vi "mod_Jakes fading profile.vi"(0 "profile length (samples)":i32=1000, 5 "sampling frequency (hz)":dbl=1.0 format="%.2f", 7 "doppler spread (hz)":dbl=1.0 format="%.2f", 9 "seed in (0xFFFFFFFF)":i32=-1 format="%.0x", 11 "error in (no error)":errorcluster, 12 "fading variance":dbl=1.0 format="%.2f", 13 "reset? (T)":bool=TRUE, 14 "number of paths":i32=1) -> (4 "fading profile":cdb[][](array[numeric]) format="%.2f", 10 "next seed":i32 format="%.0x", 15 "error out":errorcluster)   [LabVIEW 2020, in "niDMT.lvlib"]
uses:
  <vilib>/addons/Modulation/niDMT.lvlib
  <vilib>/addons/Modulation/Digital/General/subVIs/mod_Generate Bits PN Sequence.vi
  <vilib>/Analysis/7linalg.llb/Create Special Real Matrix.vi
  <vilib>/gmath/NI_Gmath.lvlib
  <vilib>/Analysis/NI_AALPro.lvlib
  <vilib>/Analysis/NI_AALBase.lvlib
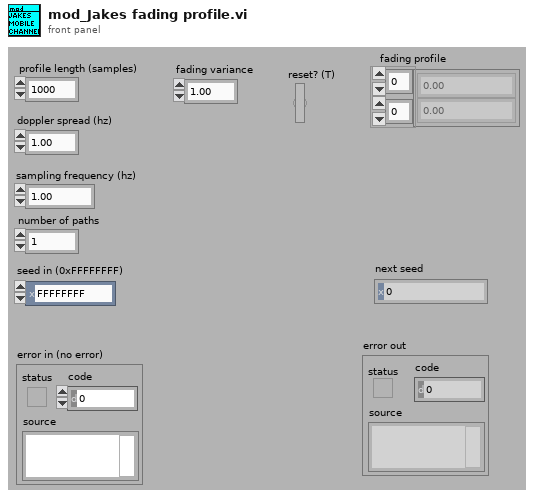
[diagram p1: front panel]
types:
  T1 = enum32{"Identity", "Diagonal", "Toepliz", "Vandermonde", "Companion"}
  T2 = typedef "NI_Matrix.lvlib/RealMatrix.ctl" = dbl[][]
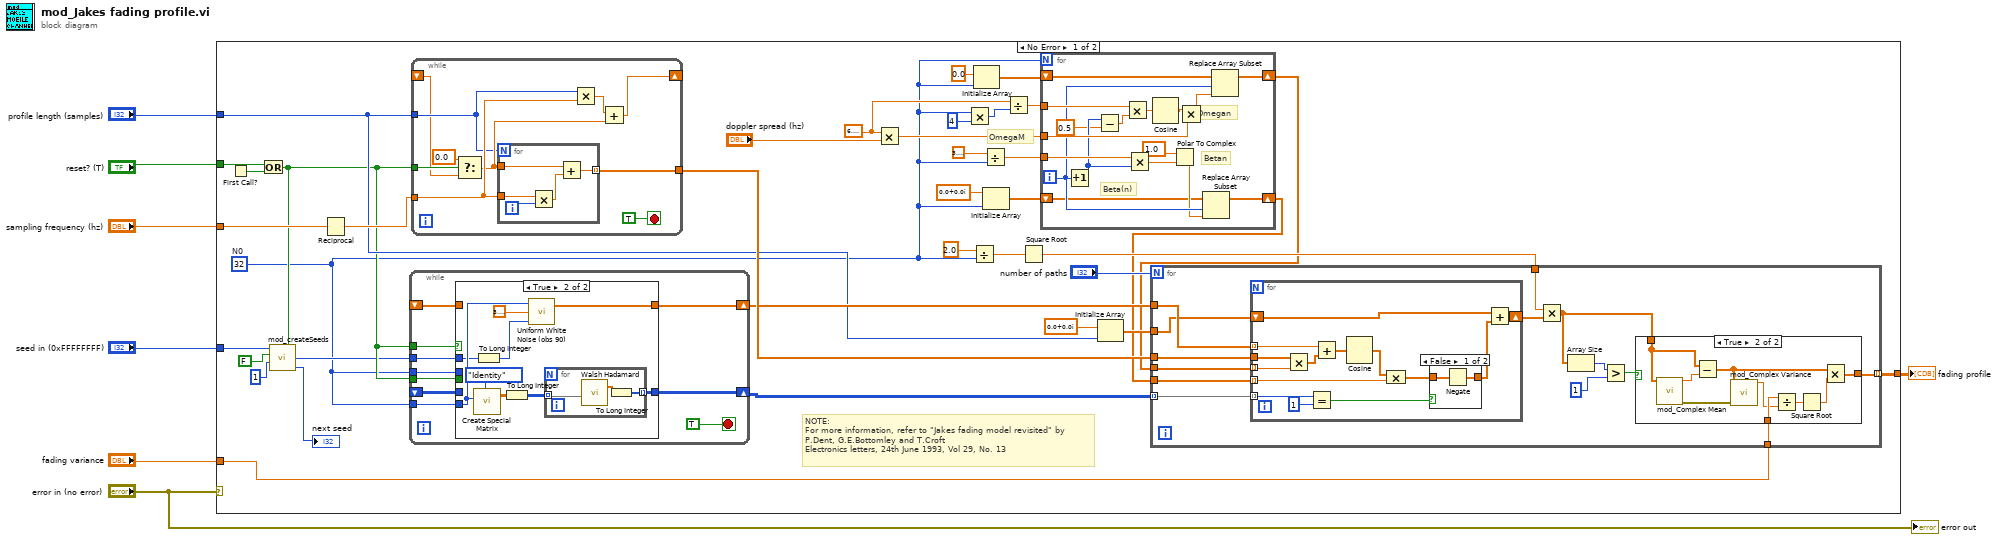
[diagram p0: block diagram]
diagram:
  n1 = case shown="No Error" "error in (no error)" {
    tunnel: [w26 _] -> w7
    tunnel: "profile length (samples)" -> [w25 _]
    tunnel: "reset? (T)" -> [w24 _]
    tunnel: "sampling frequency (hz)" -> [w23 _]
    tunnel: "seed in (0xFFFFFFFF)" -> [w21 _]
    tunnel: "fading variance" -> [w22 _]
    frame No Error {
      w15 = 6.283185307179586
      w8 = 32  # N0
      # "NOTE:\nFor more information, refer to \"Jakes fading model revisited\" by \nP.Dent, G.E.Bottomley and T.Croft\nElectronics letters, 24th June 1993, Vol 29, No. 13"
      # "OmegaM"
      n2 = First Call?() -> (First Call?: T/F=w44:bool)
      n3 = Or(x=w24, y=w44) -> (x .or. y?=w19:bool)
      n4 = call <vilib>:"mod_createSeeds.vi"("Reset? (T)"=w19, "# of seeds to create"=1, "Allow Neg if not already? (T)"=FALSE, "seed in (0xFFFFFFFF)"=w21) -> ("Next seed"=→"next seed":i32, "First Seed"=w17:i32)  [unwired: 1 out]
      n5 = Reciprocal(x=w23) -> (1/x=w43:dbl)
      n6 = while {
        tunnel: w8 -> [w49]
        tunnel: w19 -> [w53]
        shift-right: [w48] -> w35
        shift-left: _ -> [w54]
        shift-right: [w51] -> w34
        shift-left: _ -> [w50]
        tunnel: w17 -> [w47]
        tunnel: w8 -> [w46]
        tunnel: w19 -> [w45]
        stop <- TRUE stop-if-true
        n7 = case shown="True" w53 {
          tunnel: w54 -> [w55 _]
          tunnel: [w56 w63] -> w51
          tunnel: w50 -> [w56 _]
          tunnel: w49 -> [_ w62]
          tunnel: [w55 w59] -> w48
          tunnel: w47 -> [_ w61]
          tunnel: w46 -> [_ _]
          tunnel: w45 -> [_ _]
          frame False {
          }
          frame True {
            n8 = call-poly <vilib>:"Create Special Matrix.vi"("matrix type"=T1."Identity", "matrix size"=w62) -> ("Special Matrix"=w65:T2)  [unwired: 2 in, 2 out]
            n9 = To Long Integer(number=w61) -> (32bit integer=w60:i32)
            n10 = To Long Integer(number=w65) -> (32bit integer=w64:i32[][])
            n11 = call <vilib>:"Uniform White Noise (obs 90).vi"("seed"=w60, "amplitude"=3.141592653589793, "samples"=w62) -> ("uniform white noise"=w59:dbl[])  [unwired: 1 out]
            n12 = for {
              tunnel: w64 -> [w68] mode=indexing
              tunnel: [w66] -> w63 mode=indexing
              n13 = call <vilib>:"Walsh Hadamard.vi"("X"=w68) -> ("Walsh Hadamard {X}"=w67:dbl[])  [unwired: 1 out]
              n14 = To Long Integer(number=w67) -> (32bit integer=w66:i32[])
            }
          }
        }
      }
      n15 = while {
        tunnel: w19 -> [w119]
        tunnel: w43 -> [w117]
        tunnel: [w114] -> w37
        tunnel: w25 -> [w113]
        shift-right: [w111] -> _
        shift-left: _ -> [w110]
        stop <- TRUE stop-if-true
        n16 = Select(t=0.0, s=w119, f=w110) -> (s? t:f=w115:dbl)
        n17 = for {
          N: w113 -> [_]
          tunnel: w115 -> [w124]
          tunnel: w117 -> [w122]
          tunnel: [w120] -> w114 mode=indexing
          i -> [w123]
          n18 = Multiply(x=w122, y=w123) -> (x*y=w121:dbl)
          n19 = Add(x=w124, y=w121) -> (x+y=w120:dbl)
        }
        n20 = Multiply(x=w113, y=w117) -> (x*y=w116:dbl)
        n21 = Add(x=w116, y=w115) -> (x+y=w111:dbl)
      }
      n22 = Multiply(x=w15, y="doppler spread (hz)") -> (x*y=w36:dbl)
      n23 = Multiply(x=w8, y=4) -> (x*y=w33:i32)
      n24 = Divide(x=2.0, y=w8) -> (x/y=w38:dbl)
      n25 = Initialize Array(0.0 ("element"), w8) -> (w13:dbl[])
      n26 = Divide(x=3.141592653589793, y=w8) -> (x/y=w41:dbl)
      n27 = Initialize Array(cdb 0.0+0.0i ("element"), w8) -> (w10:cdb[])
      n28 = Divide(x=w15, y=w33) -> (x/y=w40:dbl)
      n29 = Square Root(x=w38) -> (sqrt(x)=w27:dbl)
      n30 = for {
        N: w8 -> [_]
        tunnel: w41 -> [w137]
        tunnel: w36 -> [w140]
        tunnel: w40 -> [w135]
        shift-right: [w131] -> w12
        shift-left: w13 -> [w130]
        shift-right: [w126] -> w9
        shift-left: w10 -> [w125]
        i -> [w128]
        # "Betan"
        # "Omegan"
        # "Beta(n)"
        n31 = Increment(x=w128) -> (x+1=w136:i32)
        n32 = Subtract(x=w136, y=0.5) -> (x-y=w133:dbl)
        n33 = Multiply(x=w135, y=w133) -> (x*y=w134:dbl)
        n34 = Multiply(x=w137, y=w136) -> (x*y=w139:dbl)
        n35 = Cosine(x=w134) -> (cos(x)=w141:dbl)
        n36 = Polar To Complex(1:w139, 2:1.0 ("r")) -> (0:w127:cdb)
        n37 = Multiply(x=w141, y=w140) -> (x*y=w129:dbl)
        n38 = Replace Array Subset(array=w125, new element=w127, index=w128) -> (w126:cdb[])
        n39 = Replace Array Subset(array=w130, new element=w129, index=w128) -> (w131:dbl[])
      }
      n40 = Initialize Array(cdb 0.0+0.0i ("element"), w25) -> (w29:cdb[])
      n41 = for {
        N: "number of paths" -> [_]
        tunnel: w35 -> [w80]
        tunnel: w37 -> [w81]
        tunnel: w12 -> [w82]
        tunnel: w9 -> [w79]
        tunnel: w34 -> [w78] mode=indexing
        tunnel: w29 -> [w77]
        tunnel: [w75] -> w26 mode=indexing
        tunnel: w22 -> [w76]
        tunnel: w27 -> [w74]
        n42 = for {
          tunnel: w82 -> [w105] mode=indexing
          tunnel: w81 -> [w106]
          tunnel: w80 -> [w103] mode=indexing
          tunnel: w79 -> [w100] mode=indexing
          shift-right: [w93] -> w73
          shift-left: w77 -> [w99]
          tunnel: w78 -> [w98] mode=indexing
          n43 = Multiply(x=w106, y=w105) -> (x*y=w104:dbl[])
          n44 = Equal?(x=w98, y=1) -> (x = y?=w96:bool)
          n45 = Add(x=w103, y=w104) -> (x+y=w102:dbl[])
          n46 = Cosine(x=w102) -> (cos(x)=w101:dbl[])
          n47 = Compound Arithmetic op=MULTIPLY(w101, w100) -> (w95:cdb[])
          n48 = case shown="False" w96 {
            tunnel: w95 -> [w108 w109]
            tunnel: [w107 w109] -> w94
            frame False {
              n49 = Negate(x=w108) -> (-x=w107:cdb[])
            }
            frame True {
            }
          }
          n50 = Add(x=w99, y=w94) -> (x+y=w93:cdb[])
        }
        n51 = Multiply(x=w74, y=w73) -> (x*y=w72:cdb[])
        n52 = Array Size(array=w72) -> (size(s)=w71:i32)
        n53 = Greater?(x=w71, y=1) -> (0:w69:bool)
        n54 = case shown="True" w69 {
          tunnel: w76 -> [_ w92]
          tunnel: [w83 w88] -> w75
          tunnel: w72 -> [w83 w85]
          frame False {
          }
          frame True {
            n55 = call <vilib>:"mod_Complex Mean.vi"("Signal In"=w85) -> ("Mean"=w87:cdb, "error out"=w84:errorcluster)  [unwired: 1 in, 12 out]
            n56 = Subtract(x=w85, y=w87) -> (x-y=w86:cdb[])
            n57 = call <vilib>:"mod_Complex Variance.vi"("Signal In"=w86, "error in (no error)"=w84) -> ("Variance"=w91:dbl)  [unwired: 13 out]
            n58 = Divide(x=w92, y=w91) -> (x/y=w90:dbl)
            n59 = Square Root(x=w90) -> (sqrt(x)=w89:dbl)
            n60 = Multiply(x=w86, y=w89) -> (x*y=w88:cdb[])
          }
        }
      }
    }
    frame Error {
    }
  }
  "fading profile" <- w7
  "error out" <- "error in (no error)"
